vi "Pairing Lines to Table.vi"(8 "error in (no error)":errorcluster, 10 "Pairing Lines":T1[](array[typedef])) -> (0 "error out":errorcluster, 1 "Disabled Items":i32[](array[numeric]), 2 "Pairing Table":string[][](array[string]))   [LabVIEW 2015, in "E2E Tag Exchange editor node.lvclass"]
uses:
  E2E Tag Exchange editor node.lvclass
  Pairing Details Line.ctl
  module/configuration/Runtime Implementation.ctl
  module/configuration/E2E Tag Exchange configuration.lvclass
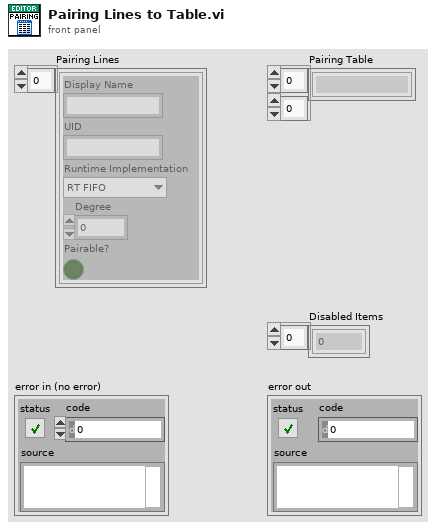
[diagram p1: front panel]
types:
  T1 = typedef "E2E Tag Exchange editor node.lvclass/Pairing Details Line.ctl" = cluster{"Display Name":string, "UID":string, "Runtime Implementation":T2, "Degree":i32, "Pairable?":bool}
  T2 = typedef "E2E Tag Exchange configuration.lvclass/Runtime Implementation.ctl" = enum16{"RT FIFO", "UDP"}
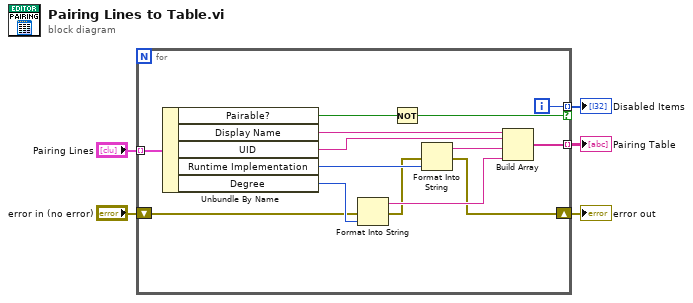
[diagram p0: block diagram]
diagram:
  n1 = for {
    tunnel: "Pairing Lines" -> [w19] mode=indexing
    shift-right: [w11] -> w4
    shift-left: "error in (no error)" -> [w10]
    tunnel: [w9] -> w3 mode=indexing
    tunnel: [w8] -> w1 mode=indexing if=w6
    i -> [w8]
    n2 = Unbundle By Name(w19) -> ("Pairable?"=w7:bool, "Display Name"=w16:string, "UID"=w15:string, "Runtime Implementation"=w17:T2, "Degree"=w18:i32)
    n3 = Format Into String(error in=w10, w18) -> (resulting string=w13:string, error out=w12:errorcluster)  [unwired: 2 in]
    n4 = Not(x=w7) -> (.not. x?=w6:bool)
    n5 = Format Into String(error in=w12, w17) -> (resulting string=w14:string, error out=w11:errorcluster)  [unwired: 2 in]
    n6 = Build Array(w16, w15, w14, w13) -> (w9:string[])
  }
  "error out" <- w4
  "Pairing Table" <- w3
  "Disabled Items" <- w1
